vi "Calculate Mean Std.vi"(8 "error in (no error)":errorcluster, 11 "Display Image in":refnum<class "Display Image.lvclass">) -> (0 "error out":errorcluster, 3 "Display Image out":refnum<class "Display Image.lvclass">)   [LabVIEW 2018, in "Display Image.lvclass"]
doc: "This VI calculates the mean and the standard deviation of the image."
uses:
  Display Image.lvclass
  Display Image.lvclass/Display Image.ctl
  <vilib>/Analysis/NI_AALBase.lvlib
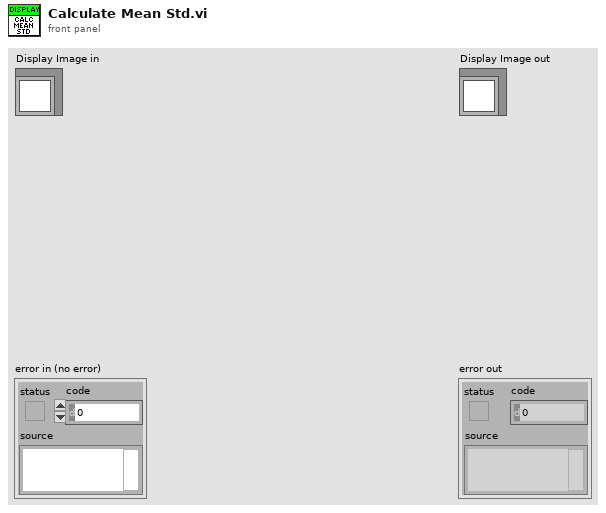
[diagram p1: front panel]
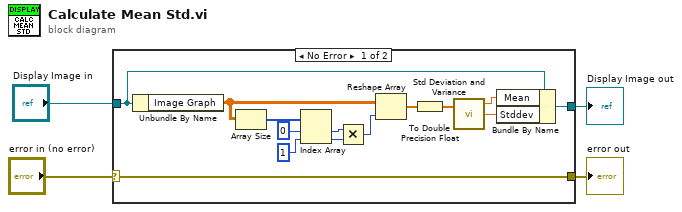
[diagram p0: block diagram]
diagram:
  n1 = case shown="No Error" "error in (no error)" {
    selector: "error in (no error)" -> [w18 w20]
    tunnel: [w18 w20] -> w3
    tunnel: [w5 w19] -> w1
    tunnel: "Display Image in" -> [w6 w19]
    frame No Error {
      n2 = Unbundle By Name(w6) -> ("Image Graph"=w11:dbl[][])
      n3 = Array Size(array=w11) -> (size(s)=w17:i32[])
      n4 = Index Array(array=w17, index #1=0 ("index"), index #2=1 ("index")) -> (element #1=w13:i32, element #2=w14:i32)
      n5 = Multiply(x=w13, y=w14) -> (x*y=w12:i32)
      n6 = Reshape Array(w11, w12) -> (w10:dbl[])
      n7 = To Double Precision Float(number=w10) -> (double precision float=w9:dbl[])
      n8 = call <vilib>:"Std Deviation and Variance.vi"("X"=w9) -> ("mean"=w7:dbl, "standard deviation"=w8:dbl)  [unwired: 1 in, 1 out]
      n9 = Bundle By Name(cluster=w6, "Mean"=w7, "Stddev"=w8) -> (w5:refnum<class "Display Image.lvclass">)
    }
    frame Error {
    }
  }
  "error out" <- w3
  "Display Image out" <- w1
